vi "Get UUT Test Results.vi"(0 "reference in":refnum<class "UUT.lvclass">, 7 "error in (no error)":errorcluster) -> (13 "Pull Passed":bool, 15 "Pull Std Dev (lb)":dbl, 17 "Pull Average (lb)":dbl, 18 "Test Results All":T1, 19 "Pull Values (lb)":dbl[](array[numeric]), 20 "reference out":refnum<class "UUT.lvclass">, 21 "Test Time":timestamp, 22 "Number of Trials":u32, 23 "Push Values (lb)":dbl[](array[numeric]), 24 "Push Average (lb)":dbl, 25 "Push Std Dev (lb)":dbl, 26 "Push Passed":bool, 27 "error out":errorcluster)   [LabVIEW 2017, in "UUT.lvclass"]
uses:
  UUT.lvclass
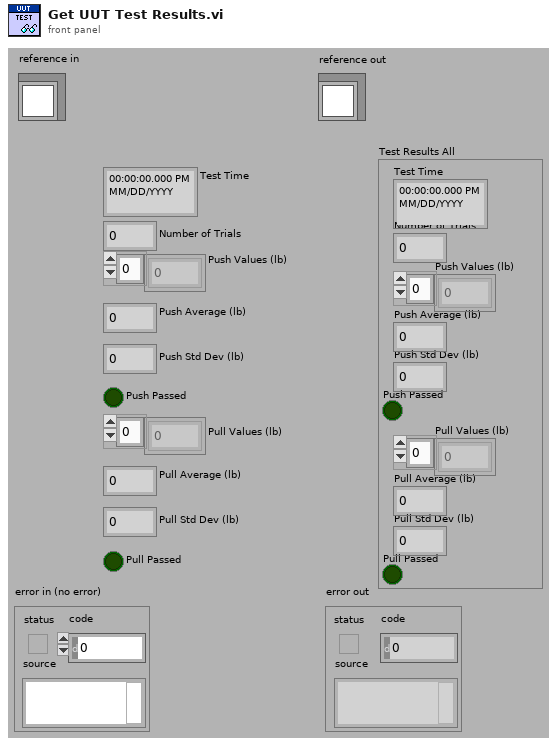
[diagram p1: front panel]
types:
  T1 = cluster{"Test Time":timestamp, "Number of Trials":u32, "Push Values (lb)":dbl[], "Push Average (lb)":dbl, "Push Std Dev (lb)":dbl, "Push Passed":bool, "Pull Values (lb)":dbl[], "Pull Average (lb)":dbl, "Pull Std Dev (lb)":dbl, "Pull Passed":bool}
  T2 = typedef "UUT.lvclass/ObjectAttributes.ctl" = cluster{"UUT Info":cluster{"Part Number":string, "Lower Push Limit (lb)":dbl, "Upper Push Limit (lb)":dbl, "Lower Pull Limit (lb)":dbl, "Upper Pull Limit (lb)":dbl, "Push Position (mm)":dbl, "Pull Position (mm)":dbl}, "Test Results":cluster{"Test Time":timestamp, "Number of Trials":u32, "Push Values (lb)":dbl[], "Push Average (lb)":dbl, "Push Std Dev (lb)":dbl, "Push Passed":bool, "Pull Values (lb)":dbl[], "Pull Average (lb)":dbl, "Pull Std Dev (lb)":dbl, "Pull Passed":bool}}
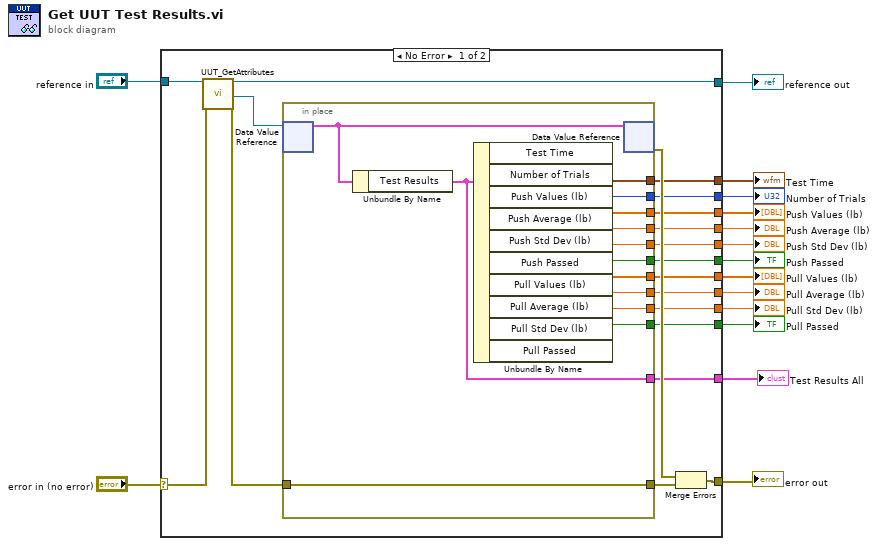
[diagram p0: block diagram]
diagram:
  n1 = case shown="No Error" "error in (no error)" {
    selector: "error in (no error)" -> [w33 w49]
    tunnel: [w31 w49] -> w14
    tunnel: [w32 w48] -> w12
    tunnel: "reference in" -> [w34 w48]
    tunnel: [w26 _] -> w11
    tunnel: [w25 _] -> w10
    tunnel: [w24 _] -> w9
    tunnel: [w23 _] -> w8
    tunnel: [w22 _] -> w7
    tunnel: [w21 _] -> w6
    tunnel: [w20 _] -> w5
    tunnel: [w19 _] -> w4
    tunnel: [w18 _] -> w3
    tunnel: [w17 _] -> w2
    tunnel: [w16 _] -> w1
    frame No Error {
      n2 = call "UUT_GetAttributes.vi"("reference in"=w34, "error in (no error)"=w33) -> ("reference out"=w32:refnum<class "UUT.lvclass">, "DataRef"=w30:refnum<data-value>, "error out"=w29:errorcluster)  [unwired: 14 in, 1 out]
      n3 = in-place {
        in-place-border: w29 -> [w47]
        in-place-border: [w47] -> w28
        in-place-border: [w45] -> w26
        in-place-border: [w44] -> w25
        in-place-border: [w43] -> w24
        in-place-border: [w42] -> w23
        in-place-border: [w41] -> w22
        in-place-border: [w40] -> w21
        in-place-border: [w39] -> w20
        in-place-border: [w38] -> w19
        in-place-border: [w37] -> w18
        in-place-border: [w36] -> w17
        in-place-border: [w35] -> w16
        n4 = in-place-dvr #1(w30) -> (w46:T2)  [unwired: 1 out]
        n5 = Unbundle By Name(w46) -> ("Test Results"=w35:T1)
        n6 = Unbundle By Name(w35) -> ("Test Time"=w36:timestamp, "Number of Trials"=w37:u32, "Push Values (lb)"=w38:dbl[], "Push Average (lb)"=w39:dbl, "Push Std Dev (lb)"=w40:dbl, "Push Passed"=w41:bool, "Pull Values (lb)"=w42:dbl[], "Pull Average (lb)"=w43:dbl, "Pull Std Dev (lb)"=w44:dbl, "Pull Passed"=w45:bool)
        n7 = in-place-dvr #1(w46) -> (w27:errorcluster)  [unwired: 1 out]
      }
      n8 = Merge Errors(w27, w28) -> (w31:errorcluster)
    }
    frame Error {
    }
  }
  "error out" <- w14
  "reference out" <- w12
  "Test Time" <- w2
  "Number of Trials" <- w3
  "Push Values (lb)" <- w4
  "Push Average (lb)" <- w5
  "Push Std Dev (lb)" <- w6
  "Push Passed" <- w7
  "Pull Values (lb)" <- w8
  "Pull Average (lb)" <- w9
  "Pull Std Dev (lb)" <- w10
  "Pull Passed" <- w11
  "Test Results All" <- w1
